vi "OutputLimeLight.vi"   [LabVIEW 2023]
doc: "This VI sends commands to the LimeLight camera."
uses:
  d59908ad-6d9d-4661-9054-5e2e0c0c3a4d.vi
  3ff4727c-c1c2-4146-b5e3-c96c6bd190a8.vi
  9228b5aa-8b6f-4f32-b857-10cfa681045f.vi
  a4c4c9eb-852e-4134-b059-2c269de838ae.vi
  bed327a2-98d3-4965-916e-7305edcf582b.vi
  9959ab12-4f3e-4c63-8bb4-e3e2fa624083.vi
  d59908ad-6d9d-4661-9054-5e2e0c0c3a4d.vi/77c742ae-e671-49bb-a825-a6e8cebc9f63.vi
  3ff4727c-c1c2-4146-b5e3-c96c6bd190a8.vi/77c742ae-e671-49bb-a825-a6e8cebc9f63.vi
  9228b5aa-8b6f-4f32-b857-10cfa681045f.vi/77c742ae-e671-49bb-a825-a6e8cebc9f63.vi
  a4c4c9eb-852e-4134-b059-2c269de838ae.vi/77c742ae-e671-49bb-a825-a6e8cebc9f63.vi
  bed327a2-98d3-4965-916e-7305edcf582b.vi/77c742ae-e671-49bb-a825-a6e8cebc9f63.vi
  9959ab12-4f3e-4c63-8bb4-e3e2fa624083.vi/77c742ae-e671-49bb-a825-a6e8cebc9f63.vi
  GlobalPoseAndTargeting.vi
  GlobalMiscellaneous.vi
  GlobalDriverStationData.vi
  Timer.vi
  <vilib>/Rock Robotics/Network Tables/NT Write Value.vi
  <vilib>/Rock Robotics/Network Tables/NT Write Number.vi
types:
  T1 = enum16{"Side-by-Side", "PiP Main", "PiP Secondary"}
  T2 = enum16{"Boot Up", "Camera Override", "AprilTags", "Gamepiece Tracking"}
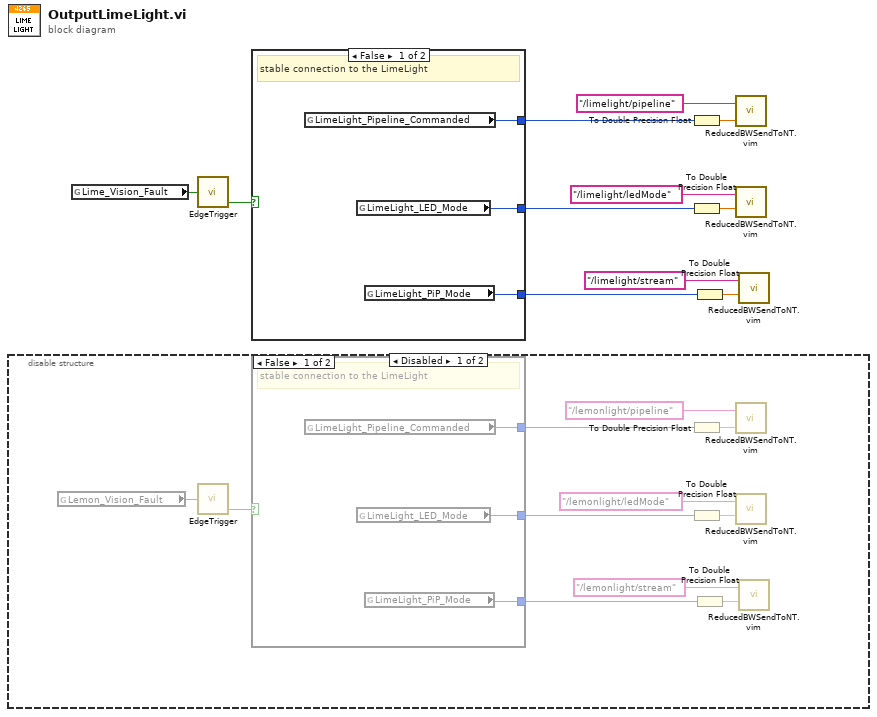
[diagram p0: block diagram]
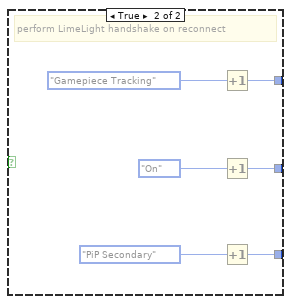
[diagram p2: hidden frame]
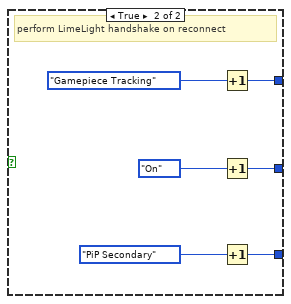
[diagram p4: hidden frame]
diagram:
  n1 = disable-structure shown="Disabled" {
    frame Disabled {
      n2 = global read "GlobalPoseAndTargeting.vi" "Lemon_Vision_Fault"() -> (w15:bool)
      n3 = call "EdgeTrigger.vi"("Input Signal"=w15) -> ("Falling Edge Trigger"=w16:bool)  [unwired: 2 out]
      n4 = case shown="False" w16 {
        tunnel: [w25 w28] -> w14
        tunnel: [w24 w27] -> w13
        tunnel: [w23 w26] -> w12
        frame False {
          # "stable connection to the LimeLight"
          n5 = global read "GlobalMiscellaneous.vi" "LimeLight_Pipeline_Commanded"() -> (w25:T2)
          n6 = global read "GlobalMiscellaneous.vi" "LimeLight_LED_Mode"() -> (w24:enum16{"Pipeline Setting", "Off", "Blink", "On"})
          n7 = global read "GlobalMiscellaneous.vi" "LimeLight_PiP_Mode"() -> (w23:T1)
        }
        frame True {
          # "perform LimeLight handshake on reconnect"
          n8 = Increment(x=T2."Gamepiece Tracking" ("LimeLight_Pipeline_Commanded")) -> (x+1=w28:T2)
          n9 = Increment(x=enum16{"Pipeline Setting", "Off", "Blink", "On"}."On" ("LimeLight_LED_Mode")) -> (x+1=w27:enum16{"Pipeline Setting", "Off", "Blink", "On"})
          n10 = Increment(x=T1."PiP Secondary" ("LimeLight_PiP_Mode")) -> (x+1=w26:T1)
        }
      }
      n11 = To Double Precision Float(number=w14) -> (double precision float=w19:dbl)
      n12 = To Double Precision Float(number=w13) -> (double precision float=w17:dbl)
      n13 = To Double Precision Float(number=w12) -> (double precision float=w21:dbl)
      n14 = call "ReducedBWSendToNT.vim"("Value In"=w19, "NT Name"="/lemonlight/pipeline" ("Name")) -> ()  [unwired: 1 out]
      n15 = call "ReducedBWSendToNT.vim"("Value In"=w17, "NT Name"="/lemonlight/ledMode" ("Name")) -> ()  [unwired: 1 out]
      n16 = call "ReducedBWSendToNT.vim"("Value In"=w21, "NT Name"="/lemonlight/stream" ("Name")) -> ()  [unwired: 1 out]
    }
    frame Enabled {
    }
  }
  n17 = global read "GlobalPoseAndTargeting.vi" "Lime_Vision_Fault"() -> (w5:bool)
  n18 = call "EdgeTrigger.vi"("Input Signal"=w5) -> ("Falling Edge Trigger"=w4:bool)  [unwired: 2 out]
  n19 = case shown="False" w4 {
    tunnel: [w34 w37] -> w3
    tunnel: [w33 w36] -> w2
    tunnel: [w32 w35] -> w1
    frame False {
      # "stable connection to the LimeLight"
      n20 = global read "GlobalMiscellaneous.vi" "LimeLight_Pipeline_Commanded"() -> (w34:T2)
      n21 = global read "GlobalMiscellaneous.vi" "LimeLight_LED_Mode"() -> (w33:enum16{"Pipeline Setting", "Off", "Blink", "On"})
      n22 = global read "GlobalMiscellaneous.vi" "LimeLight_PiP_Mode"() -> (w32:T1)
    }
    frame True {
      # "perform LimeLight handshake on reconnect"
      n23 = Increment(x=T2."Gamepiece Tracking" ("LimeLight_Pipeline_Commanded")) -> (x+1=w37:T2)
      n24 = Increment(x=enum16{"Pipeline Setting", "Off", "Blink", "On"}."On" ("LimeLight_LED_Mode")) -> (x+1=w36:enum16{"Pipeline Setting", "Off", "Blink", "On"})
      n25 = Increment(x=T1."PiP Secondary" ("LimeLight_PiP_Mode")) -> (x+1=w35:T1)
    }
  }
  n26 = To Double Precision Float(number=w3) -> (double precision float=w9:dbl)
  n27 = To Double Precision Float(number=w2) -> (double precision float=w11:dbl)
  n28 = To Double Precision Float(number=w1) -> (double precision float=w7:dbl)
  n29 = call "ReducedBWSendToNT.vim"("Value In"=w9, "NT Name"="/limelight/pipeline" ("Name")) -> ()  [unwired: 1 out]
  n30 = call "ReducedBWSendToNT.vim"("Value In"=w11, "NT Name"="/limelight/ledMode" ("Name")) -> ()  [unwired: 1 out]
  n31 = call "ReducedBWSendToNT.vim"("Value In"=w7, "NT Name"="/limelight/stream" ("Name")) -> ()  [unwired: 1 out]
